vi "Scrape Screenpops.vi"(8 "error in":errorcluster, 9 "UI":refnum<queue>, 11 "SR number list in":i32[](array[numeric])) -> (0 "error out":errorcluster, 3 "sr clusters out":T2[](array[typedef]) {"Creation Date" format="%<%x>T"; "Last Updated" format="%<%x>T"})   [LabVIEW 2018]
uses:
  Type Defs/SR Cluster.ctl
  Type Defs/SR Status.ctl
  Type Defs/SR Note Cluster.ctl
  Support/Message Queue/Message Cluster.ctl
  Support/Message Queue/Enqueue Message (Single).vi
  <vilib>/httpClient/LabVIEWHTTPClient.lvlib
  Support/Message Queue/Message Queue.lvlib
panel:
  out "body":string
  out "sr notes array out":T1[][](array[typedef]) {"Note Date" format="%<%x >T"}
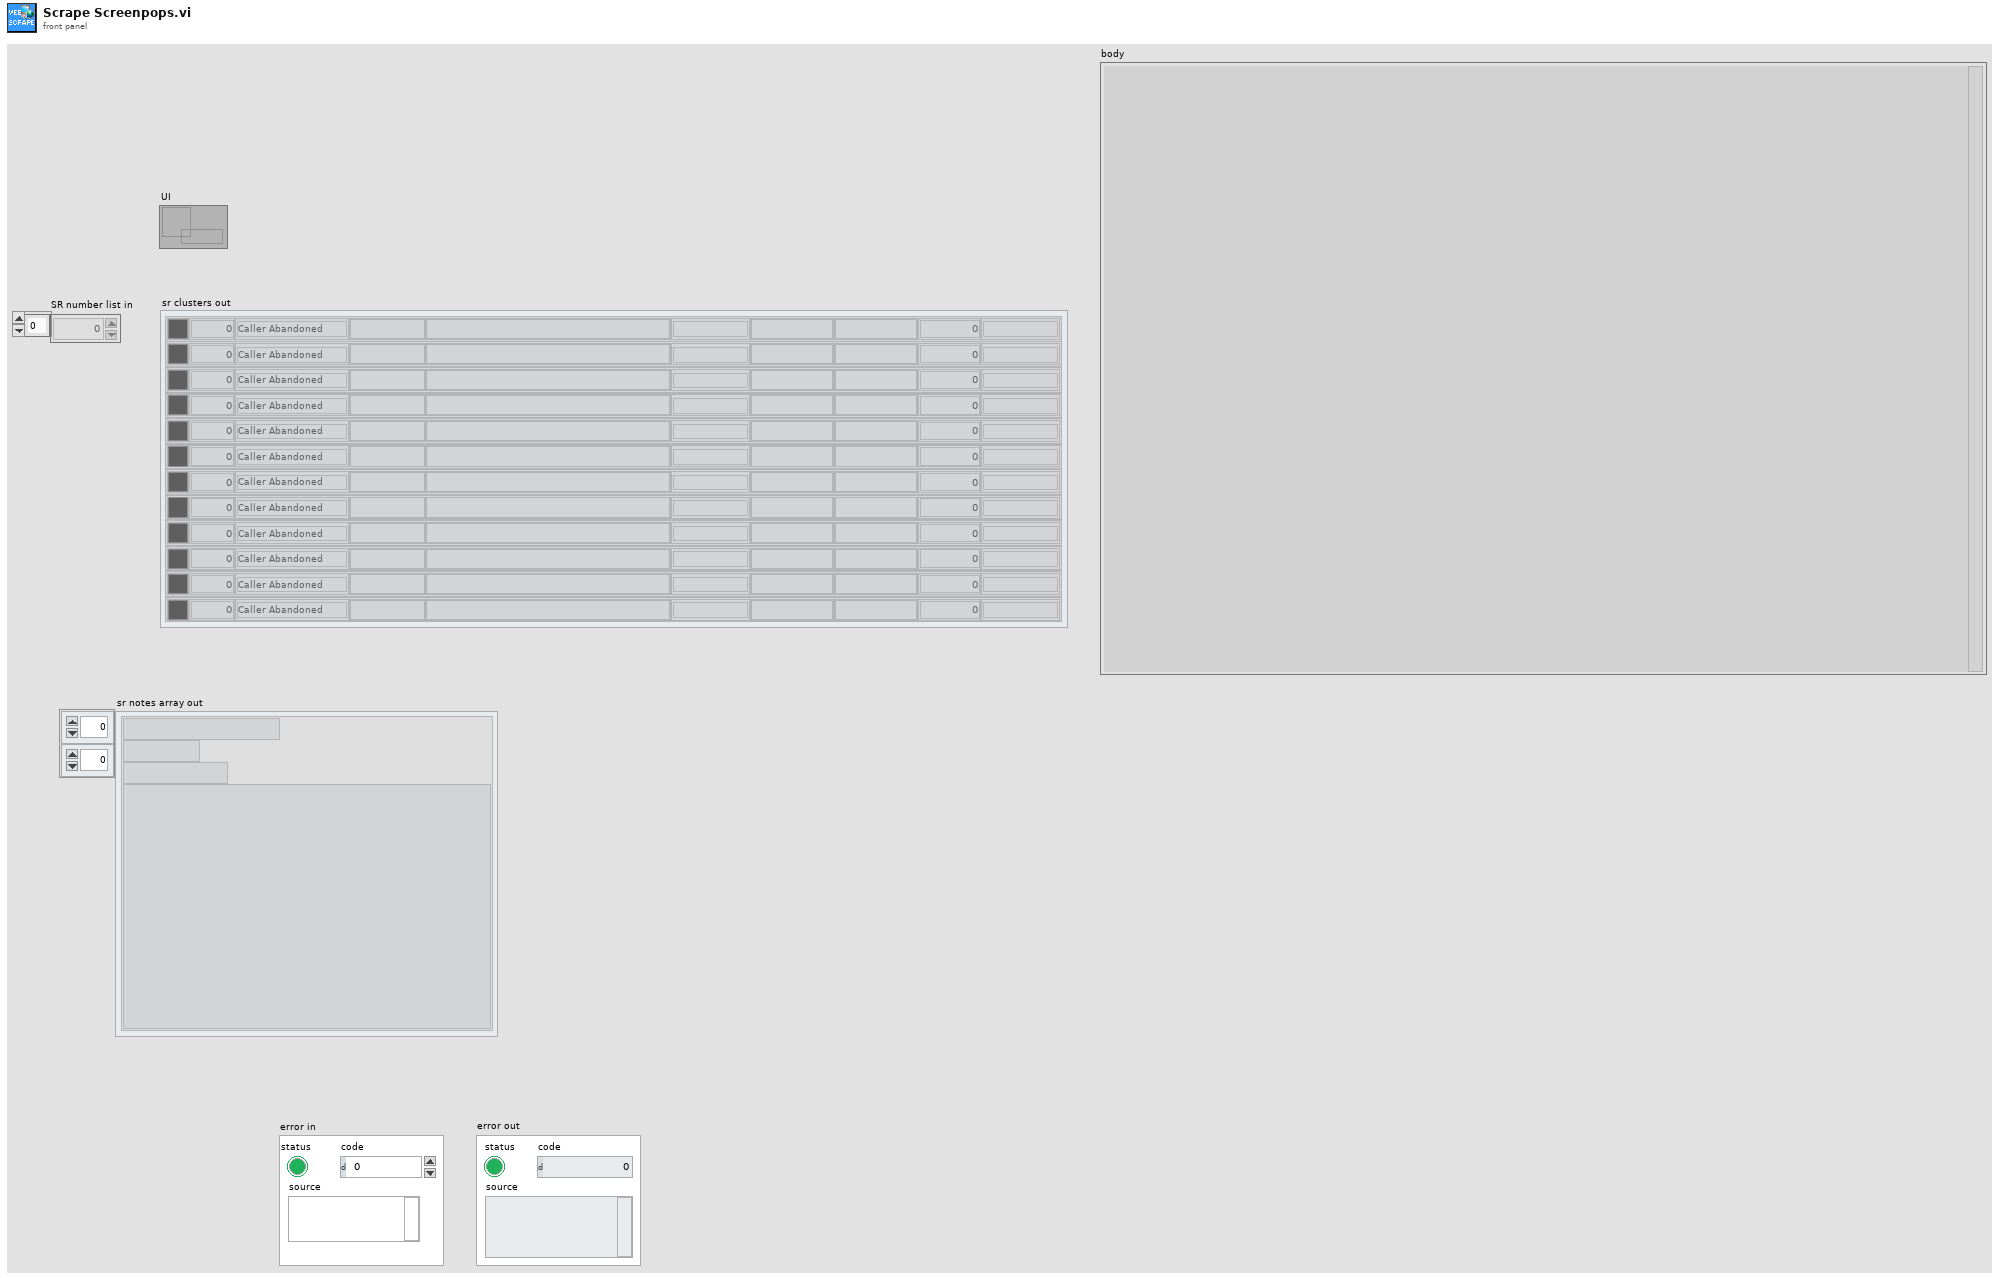
[diagram p1: front panel]
types:
  T1 = typedef "SR Note Cluster.ctl" = cluster{"Note Type":string, "Note Date":timestamp, "AE":string, "Note Text":string}
  T2 = typedef "SR Cluster.ctl" = cluster{"Color":u32, "SR Number":i32, "SR Status":T3, "Name":string, "Summary":string, "Last Updated":timestamp, "SR Type":string, "Service Level":string, "Days Open":dbl, "Creation Date":timestamp}
  T3 = typedef "SR Status.ctl" = enum16{"Caller Abandoned", "Created in Error", "Expired", "Forum Resolved AE", "Forum Resolved Customer", "IN WORK", "IN WORK Collab with AES", "IN WORK Collab with PSE", "IN WORK Collab with SE", "IN WORK Customer Added Note", "IN WORK Escalation", "IN WORK Wait on Customer", "Open", "Potentially Resolved", "Presumed Resolved", "RMA Approved for Return", "Resolved", "Passed Off"}
  T4 = typedef "LabVIEWHTTPClient.lvlib/ClientHandle.ctl" = refnum<k1>
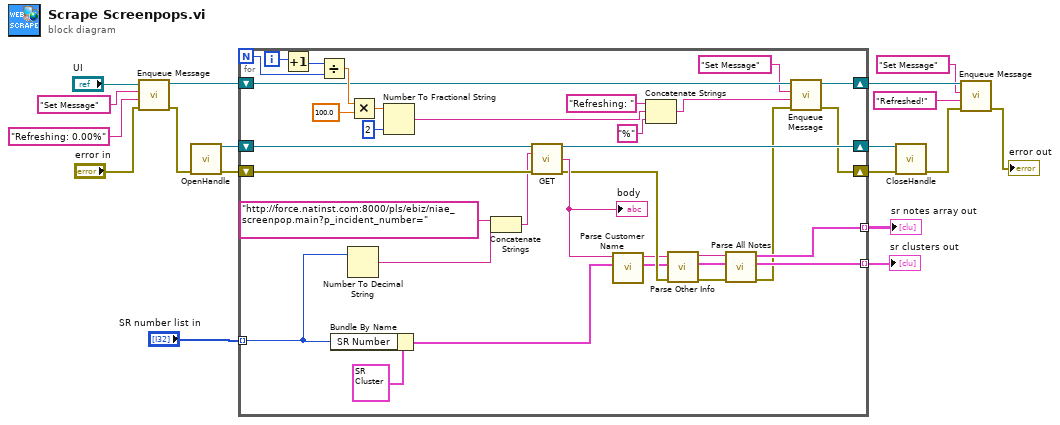
[diagram p0: block diagram]
diagram:
  n1 = call-poly "Enqueue Message.vi"("error in (no error)"="error in", "Message Data"="Refreshing: 0.00%" ("Message"), "Message"="Set Message", "Message Queue"="UI") -> ("error out"=w7:errorcluster, "dup Message Queue"=w6:refnum<queue>)  [unwired: 6 in]
  n2 = call <vilib>:"OpenHandle.vi"("error in (no error)"=w7) -> ("client handle out"=w18:T4, "error out"=w17:errorcluster)  [unwired: 13 in]
  n3 = for {
    N -> [w22]
    tunnel: "SR number list in" -> [w45] mode=indexing
    tunnel: [w47] -> w14 mode=indexing
    tunnel: [w44] -> w12 mode=indexing
    shift-right: [w35] -> w16
    shift-left: w18 -> [w52]
    shift-right: [w33] -> w15
    shift-left: w17 -> [w51]
    shift-right: [w23] -> w5
    shift-left: w6 -> [w31]
    i -> [w21]
    n4 = Increment(x=w21) -> (x+1=w20:i32)
    n5 = Divide(x=w20, y=w22) -> (x/y=w32:dbl)
    n6 = Bundle By Name(cluster=T2 {"Color"=0, "SR Number"=0, "SR Status"=enum."Caller Abandoned", "Name"="", "Summary"="", "Last Updated"=timestamp(0 s since 1904-01-01), "SR Type"="", "Service Level"="", "Days Open"=0.0, "Creation Date"=timestamp(0 s since 1904-01-01)} ("SR Cluster"), "SR Number"=w45) -> (w42:T2)
    n7 = Number To Decimal String(number=w45) -> (decimal integer string=w50:string)  [unwired: 1 in]
    n8 = Multiply(x=w32, y=100.0) -> (x*y=w26:dbl)
    n9 = Number To Fractional String(number=w26, precision (6)=i16 2) -> (F-format string=w24:string)  [unwired: 2 in]
    n10 = Concatenate Strings("http://force.natinst.com:8000/pls/ebiz/niae_screenpop.main?p_incident_number=" ("string"), w50) -> (w49:string)
    n11 = call <vilib>:"GET.vi"("client handle"=w52, "url"=w49, "error in (no error)"=w51) -> ("client handle out"=w35:T4, "body"=w43:string, "error out"=w41:errorcluster)  [unwired: 9 in, 1 out]
    "body" <- w43
    n12 = call "Parse Customer Name.vi"("SR Cluster in"=w42, "HTML text in"=w43) -> ("SR Cluster out"=w40:T2, "remaining string out"=w39:string)  [unwired: 8 in]
    n13 = Concatenate Strings("Refreshing: " ("string"), w24, "%" ("string")) -> (w28:string)
    n14 = call "Parse Other Info.vi"("error in (no error)"=w41, "SR Cluster in"=w40, "remaining string in"=w39) -> ("error out"=w36:errorcluster, "SR Cluster out 2"=w37:T2, "result string"=w38:string)  [unwired: 6 in]
    n15 = call "Parse All Notes.vi"("error in (no error)"=w36, "SR Cluster in"=w37, "result string"=w38) -> ("error out"=w34:errorcluster, "SR Cluster out"=w47:T2, "Array"=w44:T1[])  [unwired: 6 in]
    n16 = call-poly "Enqueue Message.vi"("error in (no error)"=w34, "Message Data"=w28, "Message"="Set Message", "Message Queue"=w31) -> ("error out"=w33:errorcluster, "dup Message Queue"=w23:refnum<queue>)  [unwired: 6 in]
  }
  "sr clusters out" <- w14
  "sr notes array out" <- w12
  n17 = call <vilib>:"CloseHandle.vi"("client handle"=w16, "error in (no error)"=w15) -> ("error out"=w3:errorcluster)  [unwired: 13 in]
  n18 = call-poly "Enqueue Message.vi"("error in (no error)"=w3, "Message Data"="Refreshed!" ("string"), "Message"="Set Message", "Message Queue"=w5) -> ("error out"=→"error out":errorcluster)  [unwired: 6 in, 1 out]
